vi "RT Driver VI.vi"() -> ()   [LabVIEW 2010]
uses:
  <vilib>/NI Veristand/Custom Device API/Custom Device API.lvlib
  <vilib>/NI VeriStand/Custom Device API/Get Item Property (Variant).vi
  <vilib>/NI VeriStand/Custom Device API/Custom Device Channel Type.ctl
  <vilib>/Platform/TimedLoop/XDataNode/XDataNode.xnode
  <vilib>/Platform/TimedLoop/XDataNode/nitl_modes.ctl
  <vilib>/Platform/TimedLoop/XDataNode/XDNodeRunTimeDep.lvlib
  <vilib>/Platform/TimedLoop/XDataNode/wakeup.ctl
  <vilib>/Platform/TimedLoop/XDataNode/timing_clust.ctl
  <vilib>/NI Veristand/Custom Device Tools/Custom Device Utility Library/Custom Device Utility Library.lvlib
  <vilib>/NI VeriStand/Custom Device API/Custom Device Item Ref.ctl
  Configuration Data.ctl
  Real-Time System Data.ctl
  Channel Data.ctl
panel:
  in  "Device Clock":string
  in  "Channel Data (DBLs Only)":T1
  in  "Configuration Data":T2
  in  "Real-Time System Data":T3
  in  "Status Notifier":refnum<notifier>
  in  "Device Inputs FIFO":refnum<k33>
  in  "Device Outputs FIFO":refnum<k33>
  in  "Device Reference":T4 format="%.0x"
  # "Custom Device Template\nv1.0"
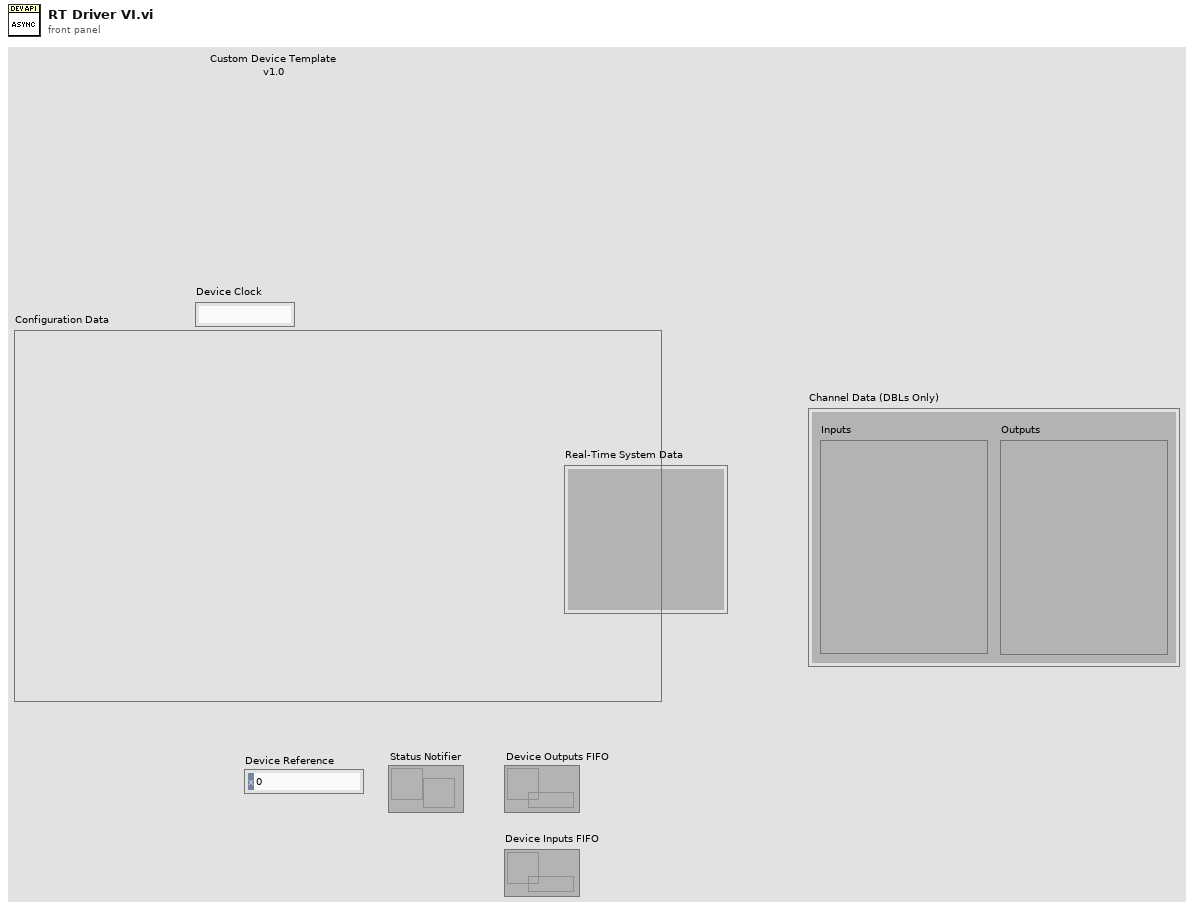
[diagram p1: front panel]
types:
  T1 = typedef "Channel Data.ctl" = cluster{"Inputs":cluster{}, "Outputs":cluster{}}
  T2 = typedef "Configuration Data.ctl" = cluster{}
  T3 = typedef "Real-Time System Data.ctl" = cluster{}
  T4 = typedef "Custom Device API.lvlib/Custom Device Item Ref.ctl" = u64
  T5 = typedef "Custom Device API.lvlib/Custom Device Channel Type.ctl" = enum16{"Input", "Output"}
  T6 = typedef "XDNodeRunTimeDep.lvlib/timing_clust.ctl" = cluster{"Expected End [f-1]":u64, "Actual End [f-1]":u64, "Finished Late? [f-1]":bool, "Expected End [i-1]":u64, "Actual End [i-1]":u64, "Finished Late? [i-1]":bool, "Expected Start [i]":u64, "Actual Start [i]":u64, "Expected Start [f]":u64, "Actual Start [f]":u64, "Source Name":string, "Structure Name":string, "Period":i64, "Deadline":i64, "Offset":i64, "Start":i64, "Priority":i32, "Timeout":i32, "Mode":T7, "Wakeup Reason":T8, "Error":errorcluster, "Source Type":string, "Secondary Source Type":string, "Global End Time":u64, "Global Start Time":u64, "Frame Duration":u64, "Iteration Duration":u64, "Assigned CPU":i32, "I/O Scan Engine Mode":u32}
  T7 = typedef "XDNodeRunTimeDep.lvlib/nitl_modes.ctl" = enum32{"No Change", "Process missed periods, maintain original phase", "Discard missed periods, maintain original phase", "Process missed periods, ignore original phase", "Discard missed periods, ignore original phase"}
  T8 = typedef "XDNodeRunTimeDep.lvlib/wakeup.ctl" = enum32{"Normal", "Aborted", "Asynchronous wakeup", "Timing source error", "Timed loop error", "Timeout"}
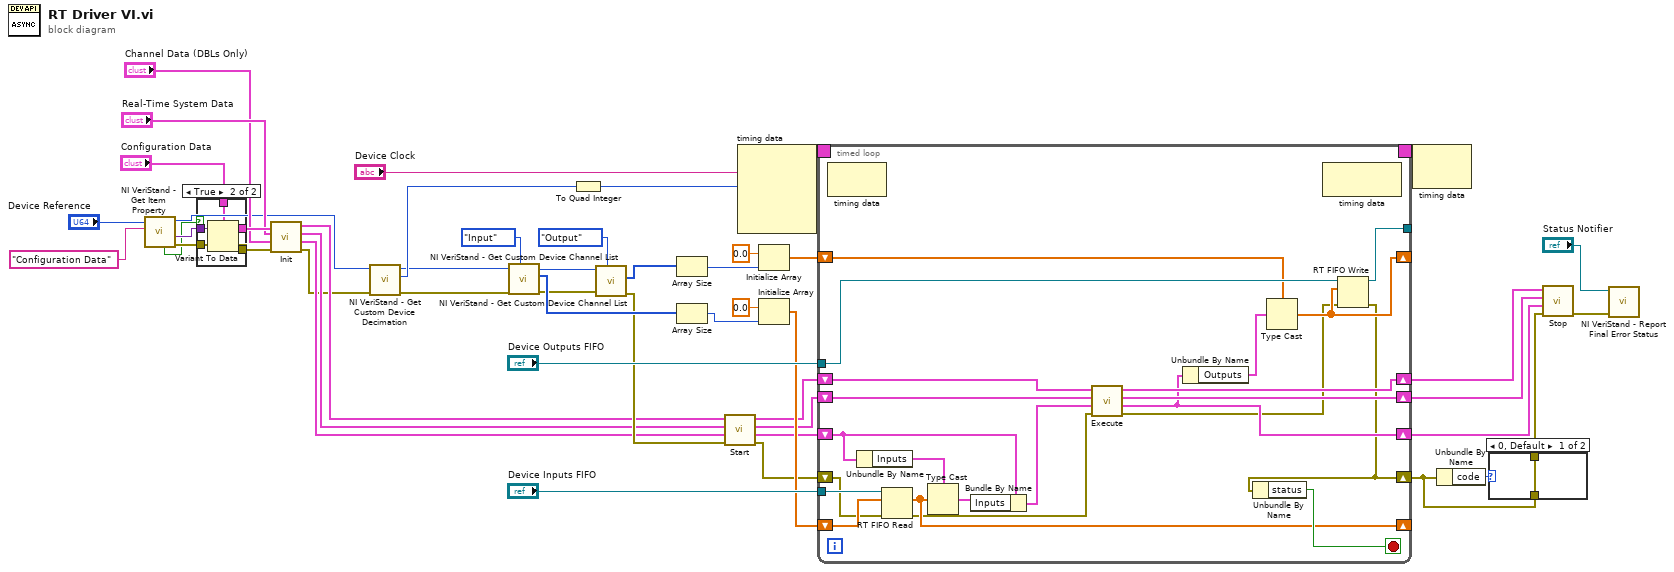
[diagram p0: block diagram]
diagram:
  n1 = call-poly <vilib>:"NI VeriStand - Get Item Property.vi"("Property Name"="Configuration Data", "Item Ref in"="Device Reference") -> ("error out"=w46:errorcluster, "Value"=w45:variant, "Item Ref out"=w14:T4, "Found?"=w6:bool)  [unwired: 6 in]
  n2 = case shown="True" w6 {
    tunnel: w46 -> [w51 w56]
    tunnel: w45 -> [_ w55]
    tunnel: "Configuration Data" -> [w50 w54]
    tunnel: [w50 w53] -> w43
    tunnel: [w51 w52] -> w42
    frame False {
    }
    frame True {
      n3 = Variant To Data(error in=w56, Variant=w55, type=w54) -> (error out=w52:errorcluster, data=w53:T2)
    }
  }
  n4 = call "Init.vi"("error in (no error)"=w42, "Channel Data (DBLs Only)"="Channel Data (DBLs Only)", "Real-Time System Data"="Real-Time System Data", "Configuration Data"=w43) -> ("error out"=w13:errorcluster, "Channel Data (DBLs Only)"=w25:T1, "Real-Time System Data"=w26:T3, "Configuration Data"=w18:T2)  [unwired: 4 in]
  n5 = call <vilib>:"NI VeriStand - Get Custom Device Decimation.vi"("error in (no error)"=w13, "Device Ref in"=w14) -> ("error out"=w8:errorcluster, "Decimation"=w12:i32, "Device Ref out"=w9:T4)  [unwired: 7 in]
  n6 = call <vilib>:"NI VeriStand - Get Custom Device Channel List.vi"("Channel Type"=Custom_Device_Channel_Type."Input", "error in (no error)"=w8, "Device Ref in"=w9) -> ("error out"=w28:errorcluster, "Specified Channel Ref List"=w38:T4[], "Device Ref out"=w40:T4)  [unwired: 6 in]
  n7 = To Quad Integer(1:w12) -> (0:w11:i64)
  n8 = call <vilib>:"NI VeriStand - Get Custom Device Channel List.vi"("Channel Type"=Custom_Device_Channel_Type."Output", "error in (no error)"=w28, "Device Ref in"=w40) -> ("error out"=w27:errorcluster, "Specified Channel Ref List"=w37:T4[])  [unwired: 6 in, 1 out]
  n9 = Array Size(array=w37) -> (size(s)=w35:i32)
  n10 = Array Size(array=w38) -> (size(s)=w36:i32)
  n11 = call "Start.vi"("error in (no error)"=w27, "Channel Data (DBLs Only)"=w25, "Real-Time System Data"=w26, "Configuration Data"=w18) -> ("error out"=w7:errorcluster, "Channel Data (DBLs Only)"=w24:T1, "Real-Time System Data"=w17:T3, "Configuration Data"=w20:T2)  [unwired: 4 in]
  n12 = node-c288("Device Clock", w11) -> (w16:T6)  [unwired: 2 in]
  n13 = Initialize Array(0.0 ("element"), w35) -> (w32:dbl[])
  n14 = Initialize Array(0.0 ("element"), w36) -> (w31:dbl[])
  n15 = timed-loop {
    tunnel: "Device Inputs FIFO" -> [w78]
    tunnel: "Device Outputs FIFO" -> [w77]
    tunnel: [w76] -> _
    shift-right: [w68] -> _
    shift-left: w32 -> [w69]
    shift-right: [w67] -> _
    shift-left: w31 -> [w74]
    shift-right: [w65] -> w23
    shift-left: w17 -> [w62]
    shift-right: [w64] -> w22
    shift-left: w24 -> [w73]
    shift-right: [w66] -> w19
    shift-left: w20 -> [w63]
    timing: w16 -> [_]
    timing-out: [_] -> w15
    shift-right: [w57] -> w2
    shift-left: w7 -> [w60]
    stop <- w75 stop-if-true
    n16 = node-c288() -> ()  [unwired: 1 in, 1 out]
    n17 = Unbundle By Name(w73) -> ("Inputs"=w72:cluster{})
    n18 = RT FIFO Read(0:w78, 1:w74, 3:w60) -> (9:w67:dbl[], 11:w59:errorcluster)  [unwired: 1 in, 3 out]
    n19 = Type Cast(type=w72, x=w67) -> (*(type *) &x=w71:cluster{})
    n20 = Bundle By Name(cluster=w73, "Inputs"=w71) -> (w61:T1)
    n21 = call "Execute.vi"("error in (no error)"=w59, "Channel Data (DBLs Only)"=w61, "Real-Time System Data"=w62, "Configuration Data"=w63) -> ("error out"=w58:errorcluster, "Channel Data (DBLs Only)"=w64:T1, "Real-Time System Data"=w65:T3, "Configuration Data"=w66:T2)  [unwired: 4 in]
    n22 = Unbundle By Name(w64) -> ("Outputs"=w70:cluster{})
    n23 = Type Cast(type=w69, x=w70) -> (*(type *) &x=w68:dbl[])
    n24 = node-c288() -> ()  [unwired: 1 in, 1 out]
    n25 = RT FIFO Write(0:w77, 1:w68, 3:w58) -> (8:w76:refnum<k33>, 11:w57:errorcluster)  [unwired: 2 in, 2 out]
    n26 = Unbundle By Name(w57) -> ("status"=w75:bool)
  }
  n27 = node-c288(w15) -> ()  [unwired: 1 out]
  n28 = Unbundle By Name(w2) -> ("code"=w3:i32)
  n29 = case shown="0, Default" w3 {
    tunnel: w2 -> [w81 _]
    tunnel: [w81 _] -> w1
    frame 0, Default {
    }
    frame -2206 {
    }
  }
  n30 = call "Stop.vi"("error in (no error)"=w1, "Channel Data (DBLs Only)"=w22, "Real-Time System Data"=w23, "Configuration Data"=w19) -> ("error out"=w5:errorcluster)  [unwired: 7 in]
  n31 = call <vilib>:"NI VeriStand - Report Final Error Status.vi"("error in (no error)"=w5, "Status Notifier"="Status Notifier") -> ()  [unwired: 1 in, 9 out]
